vi "FlatToRichnixnet_grpc_CreateSessionByRefRequest.vi"(5 "OutputClusterType":T1, 11 "InputCluster":T4) -> (3 "OutputCluster":T1)   [LabVIEW 2025, in "xnet-grpc_client.lvlib"]
uses:
  nixnet_grpc_CreateSessionByRefRequest_Flat.ctl
  nidevice_grpc_Session_Flat.ctl
  nixnet_grpc_CreateSessionMode.ctl
  nidevice_grpc_SessionInitializationBehavior.ctl
  nixnet_grpc_CreateSessionByRefRequest.ctl
  nixnet_grpc_CreateSessionByRefRequest_mode_enum/nixnet_grpc_CreateSessionByRefRequest_mode_enum.lvclass
  nidevice_grpc_Session.ctl
  xnet-grpc_client.lvlib
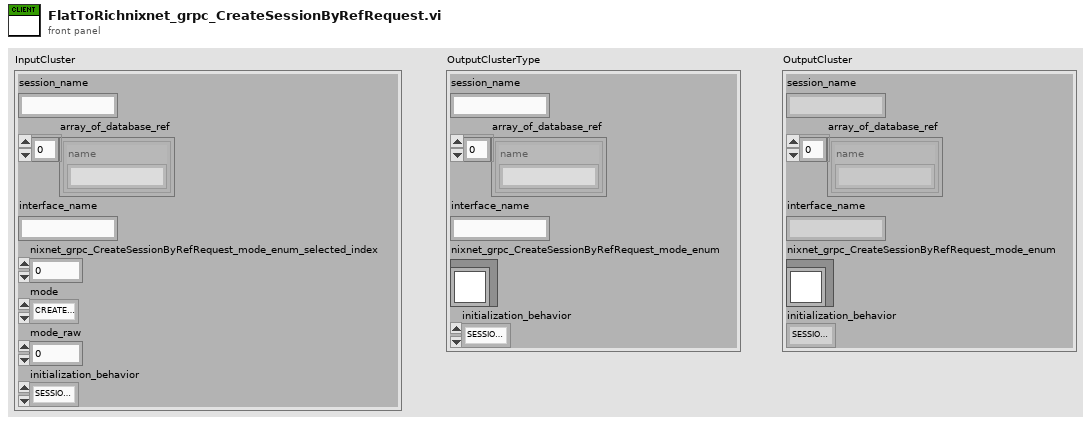
[diagram p1: front panel]
types:
  T1 = typedef "xnet-grpc_client.lvlib/nixnet_grpc_CreateSessionByRefRequest.ctl" = cluster{"session_name":string, "array_of_database_ref":T2[], "interface_name":string, "nixnet_grpc_CreateSessionByRefRequest_mode_enum":refnum<class "nixnet_grpc_CreateSessionByRefRequest_mode_enum.lvclass">, "initialization_behavior":T3}
  T2 = typedef "xnet-grpc_client.lvlib/nidevice_grpc_Session.ctl" = cluster{"name":string}
  T3 = typedef "xnet-grpc_client.lvlib/nidevice_grpc_SessionInitializationBehavior.ctl" = enum32{"SESSION_INITIALIZATION_BEHAVIOR_UNSPECIFIED", "SESSION_INITIALIZATION_BEHAVIOR_INITIALIZE_NEW", "SESSION_INITIALIZATION_BEHAVIOR_ATTACH_TO_EXISTING"}
  T4 = typedef "xnet-grpc_client.lvlib/nixnet_grpc_CreateSessionByRefRequest_Flat.ctl" = cluster{"session_name":string, "array_of_database_ref":T5[], "interface_name":string, "nixnet_grpc_CreateSessionByRefRequest_mode_enum_selected_index":i32, "mode":T6, "mode_raw":u32, "initialization_behavior":T3}
  T5 = typedef "xnet-grpc_client.lvlib/nidevice_grpc_Session_Flat.ctl" = cluster{"name":string}
  T6 = typedef "xnet-grpc_client.lvlib/nixnet_grpc_CreateSessionMode.ctl" = enum32{"CREATE_SESSION_MODE_SIGNAL_IN_SINGLE_POINT", "CREATE_SESSION_MODE_SIGNAL_IN_WAVEFORM", "CREATE_SESSION_MODE_SIGNAL_IN_XY", "CREATE_SESSION_MODE_SIGNAL_OUT_SINGLE_POINT", "CREATE_SESSION_MODE_SIGNAL_OUT_WAVEFORM", "CREATE_SESSION_MODE_SIGNAL_OUT_XY", "CREATE_SESSION_MODE_FRAME_IN_STREAM", "CREATE_SESSION_MODE_FRAME_IN_QUEUED", "CREATE_SESSION_MODE_FRAME_IN_SINGLE_POINT", "CREATE_SESSION_MODE_FRAME_OUT_STREAM", "CREATE_SESSION_MODE_FRAME_OUT_QUEUED", "CREATE_SESSION_MODE_FRAME_OUT_SINGLE_POINT", "CREATE_SESSION_MODE_SIGNAL_CONVERSION_SINGLE_POINT"}
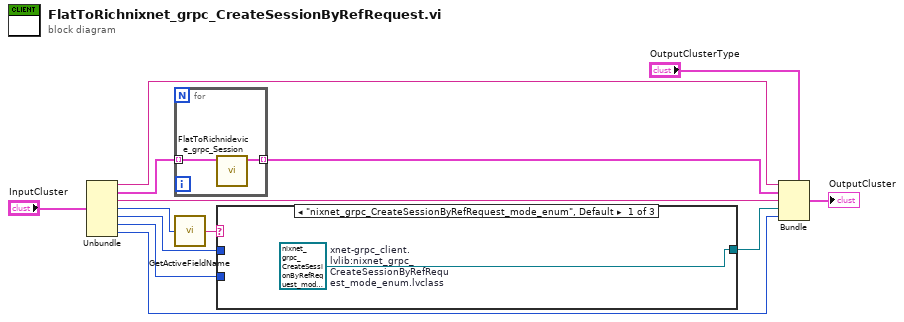
[diagram p0: block diagram]
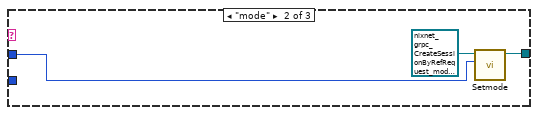
[diagram p2: hidden frame]
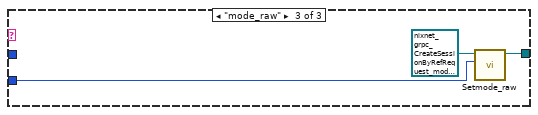
[diagram p3: hidden frame]
diagram:
  n1 = Unbundle "Unbundle"("InputCluster") -> ("session_name"=w10:string, "array_of_database_ref"=w9:T5[], "interface_name"=w7:string, "nixnet_grpc_CreateSessionByRefRequest_mode_enum_selected_index"=w6:i32, "mode"=w3:T6, "mode_raw"=w2:u32, "initialization_behavior"=w1:T3)
  n2 = for {
    tunnel: w9 -> [w15] mode=indexing
    tunnel: [w14] -> w8 mode=indexing
    n3 = call "FlatToRichnidevice_grpc_Session.vi"("InputCluster"=w15) -> ("OutputCluster"=w14:T2)  [unwired: 10 in]
  }
  n4 = call "GetActiveFieldName.vi"("protobuf index"=w6) -> ("oneof field name"=w5:string)
  n5 = case "nixnet_grpc_CreateSessionByRefRequest_mode_enum" shown="\"nixnet_grpc_CreateSessionByRefRequest_mode_enum\", Default" w5 {
    tunnel: [w16 w18 w21] -> w4
    tunnel: w3 -> [_ w19 _]
    tunnel: w2 -> [_ _ w22]
    frame "nixnet_grpc_CreateSessionByRefRequest_mode_enum", Default {
      w16 = refnum<class "nixnet_grpc_CreateSessionByRefRequest_mode_enum.lvclass"> refnum  # xnet-grpc_client.lvlib:nixnet_grpc_CreateSessionByRefRequest_mode_enum.lvclass
    }
    frame "mode" {
      n6 = call "Setmode.vi"("Set_Val"=w19, "OneOfTemplate in"=refnum<class "nixnet_grpc_CreateSessionByRefRequest_mode_enum.lvclass"> refnum) -> ("OneOfTemplate out"=w18:refnum<class "nixnet_grpc_CreateSessionByRefRequest_mode_enum.lvclass">)  [unwired: 8 in, 1 out]
    }
    frame "mode_raw" {
      n7 = call "Setmode_raw.vi"("Set_Val"=w22, "OneOfTemplate in"=refnum<class "nixnet_grpc_CreateSessionByRefRequest_mode_enum.lvclass"> refnum) -> ("OneOfTemplate out"=w21:refnum<class "nixnet_grpc_CreateSessionByRefRequest_mode_enum.lvclass">)  [unwired: 8 in, 1 out]
    }
  }
  n8 = Bundle "Bundle"(cluster="OutputClusterType", "session_name"=w10, "array_of_database_ref"=w8, "interface_name"=w7, "nixnet_grpc_CreateSessionByRefRequest_mode_enum"=w4, "initialization_behavior"=w1) -> (→"OutputCluster":T1)
